vi "Update.vi"(8 "error in (no error)":errorcluster, 11 "subpanel (abstract) in":refnum<class "subpanel (abstract).lvclass">) -> (0 "error out":errorcluster, 3 "subpanel (abstract) out":refnum<class "subpanel (abstract).lvclass">)   [LabVIEW 2023, in "GUI.lvlib" / "subpanel (abstract).lvclass"]
uses:
  subpanel (abstract).lvclass
  subpanel (abstract).lvclass/subpanel (abstract).ctl
  <vilib>/Utility/miscctls.llb/LVPositionTypeDef.ctl
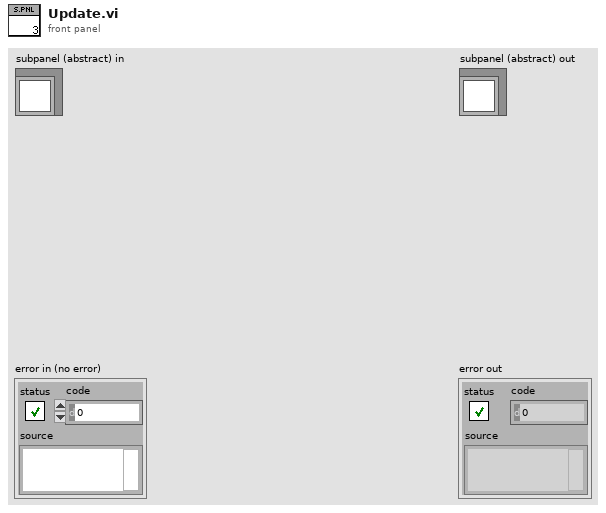
[diagram p1: front panel]
types:
  T1 = typedef "LVPositionTypeDef.ctl" = cluster{"Left":i32, "Top":i32}
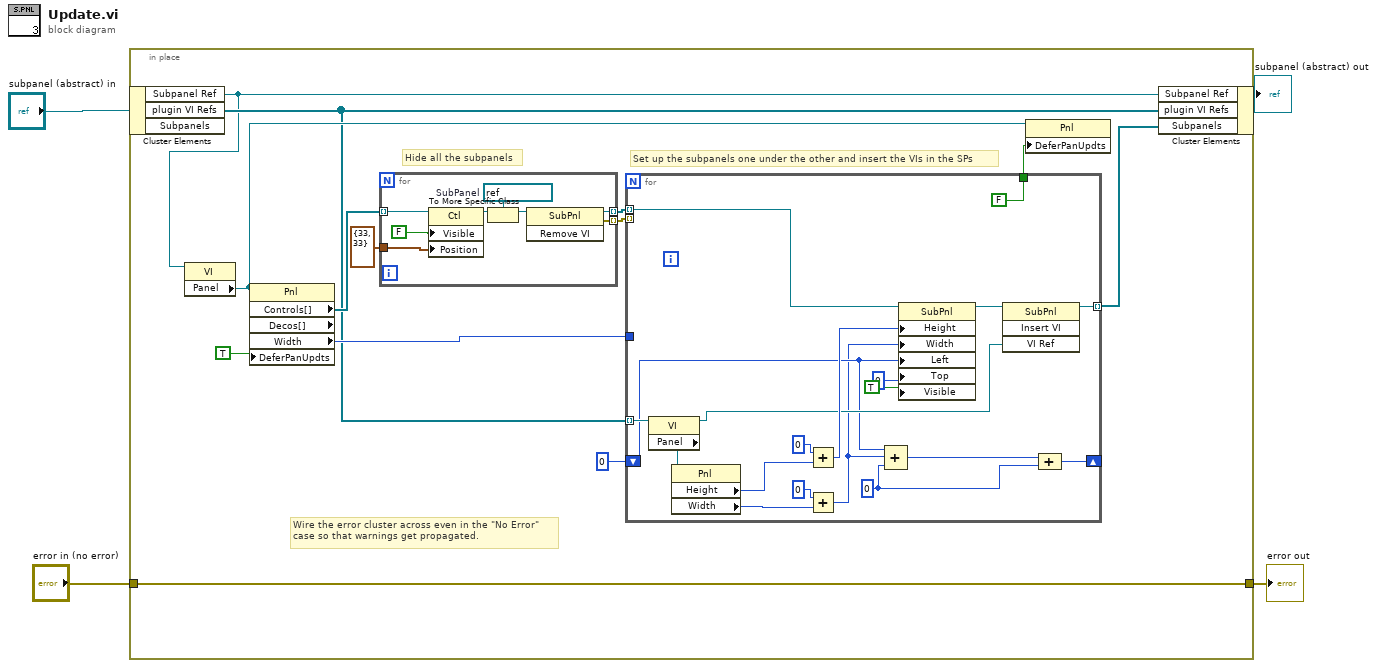
[diagram p0: block diagram]
diagram:
  n1 = in-place {
    in-place-border: "error in (no error)" -> [w17]
    in-place-border: [w17] -> w1
    # "Set up the subpanels one under the other and insert the VIs in the SPs"
    # "Hide all the subpanels"
    # "Wire the error cluster across even in the \"No Error\"\ncase so that warnings get propagated."
    n2 = in-place-cluster #1("subpanel (abstract) in") -> ("Subpanel Ref"=w5:refnum<vi>, "plugin VI Refs"=w6:refnum<vi>[])  [unwired: 1 out]
    n3 = property class="VI"(reference=w5) -> ("Panel"=w8:refnum<vi>)  [unwired: 1 in, 2 out]
    n4 = property class="Pnl" props=["Controls[]", "Decos[]", "Width", "DeferPanUpdts"](reference=w8, "DeferPanUpdts"=TRUE ("Defer Panel Updates")) -> ("Controls[]"=w14:refnum<vi>[], "Width"=w16:u32)  [unwired: 1 in, 3 out]
    n5 = for {
      tunnel: w14 -> [w25] mode=indexing
      tunnel: T1 {"Left"=33, "Top"=33} ("Position") -> [w23]
      tunnel: [w19] -> w10 mode=indexing
      tunnel: [w18] -> w9 mode=indexing
      w22 = refnum<vi> refnum  # SubPanel
      n6 = property class="Ctl"(reference=w25, "Visible"=FALSE, "Position"=w23) -> (reference out=w20:refnum<vi>)  [unwired: 1 in, 1 out]
      n7 = To More Specific Class(target class=w22, reference=w20) -> (specific class reference=w21:refnum<vi>)  [unwired: 1 in, 1 out]
      n8 = invoke class="SubPnl" method="Remove VI"(reference=w21) -> (reference out=w18:refnum<vi>, error out=w19:errorcluster)  [unwired: 2 in, 1 out]
    }
    n9 = for {
      shift-right: [w41] -> _
      shift-left: 0 -> [w28]
      tunnel: w6 -> [w31] mode=indexing
      tunnel: [w37] -> w7 mode=indexing
      tunnel: w16 -> [_]
      tunnel: [FALSE ("Defer Panel Updates")] -> w11
      tunnel: w10 -> [_] mode=indexing
      tunnel: w9 -> [w32] mode=indexing
      w42 = 0 ("value")
      n10 = property class="VI"(reference=w31) -> (reference out=w30:refnum<vi>, "Panel"=w40:refnum<vi>)  [unwired: 1 in, 1 out]
      n11 = property class="Pnl"(reference=w40) -> ("Height"=w27:u32, "Width"=w33:u32)  [unwired: 1 in, 2 out]
      n12 = Add(x=0, y=w27) -> (x+y=w39:u32)
      n13 = Add(x=u32 0, y=w33) -> (x+y=w26:u32)
      n14 = Compound Arithmetic op=ADD(w28, w26, w42) -> (w43:u32)
      n15 = property class="SubPnl"(reference=w32, "Height"=w39, "Width"=w26, "Left"=w28, "Top"=0, "Visible"=TRUE) -> (reference out=w44:refnum<vi>)  [unwired: 1 in, 1 out]
      n16 = invoke class="SubPnl" method="Insert VI"(reference=w44, "VI Ref"=w30) -> (reference out=w37:refnum<vi>)  [unwired: 2 in, 3 out]
      n17 = Compound Arithmetic op=ADD(w43, w42) -> (w41:u32)
    }
    n18 = property class="Pnl"(reference=w8, "DeferPanUpdts"=w11) -> ()  [unwired: 1 in, 2 out]
    n19 = in-place-cluster #1("Subpanel Ref"=w5, "plugin VI Refs"=w6, "Subpanels"=w7) -> (→"subpanel (abstract) out":refnum<class "subpanel (abstract).lvclass">)
  }
  "error out" <- w1
